vi "IT-M3900C List Output.vi"() -> ()   [LabVIEW 2015]
doc: "This example is used to edit the user - defined waveform function in source mode, call and implement the waveform output."
uses:
  <instrlib>/IT-M3900C/IT-M3900C.lvlib
panel:
  in  "Normal Voltage(V)":dbl min=0.0
  in  "Normal Current(A)":dbl
  in  "Serial Configuration":T1={"Baud Rate"=9600, "Parity"=0, "Data Bits"=8, "Stop Bits"=10, "Flow Control"=0} {"Flow Control" items=["None", "XON/XOFF", "RTS/CTS", "XON/XOFF & RTS/CTS", "DTR/DSR", "XON/XOFF & DTR/DSR"]; "Stop Bits" items=["1.0"=10, "1.5"=15, "2.0"=20]; "Data Bits" items=["7"=7, "8"=8]; "Parity" items=["None", "Odd", "Even", "Mark", "Space"]; "Baud Rate" items=["300"=300, "600"=600, "1200"=1200, "2400"=2400, "4800"=4800, "9600"=9600, "19200"=19200, "38400"=38400, "57600"=57600, "115200"=115200]}
  in  "Type":u16(ring) items=["Current", "Voltage"]
  in  "Save File(1-10)":i32=1 min=1 max=10
  in  "Terminate Type":u16(ring) items=["Normal", "Last", "Off"]
  in  "Repeat":i32 min=0
  in  "Slew":dbl[](array[numeric]) min=0.0
  in  "Dwell(S)":dbl[](array[numeric]) min=0.0
  in  "Level(V/A/W/ohm)":dbl[](array[numeric]) min=0.0
  in  "VISA resource name":refnum<visa-resource-name>
  # "List Function"
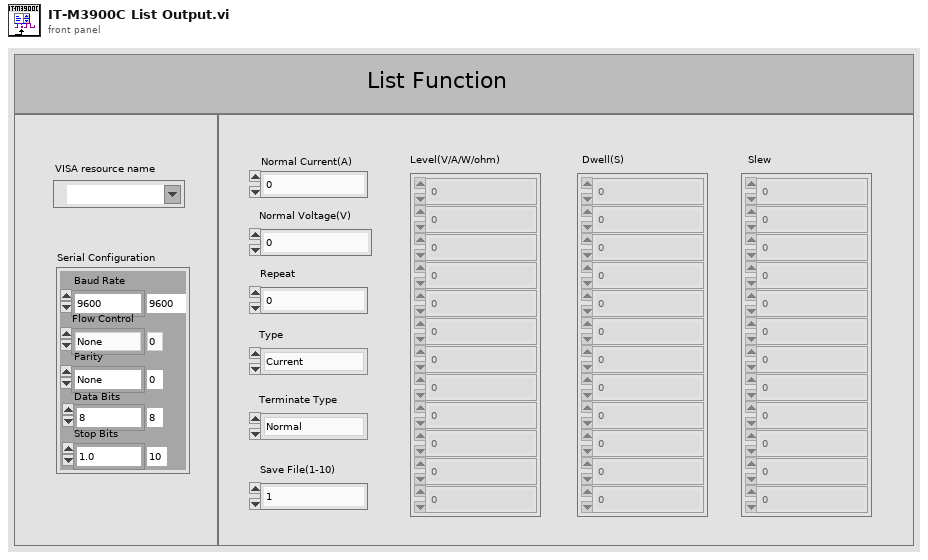
[diagram p1: front panel]
types:
  T1 = cluster{"Baud Rate":u32, "Parity":u16, "Data Bits":u16, "Stop Bits":u16, "Flow Control":u16}
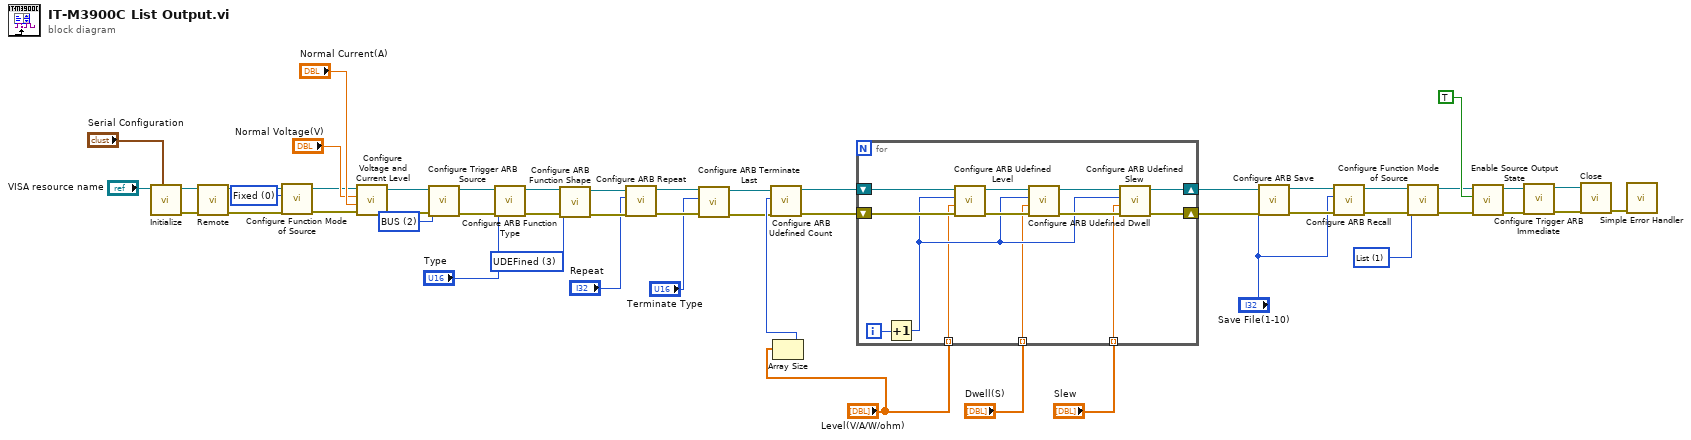
[diagram p0: block diagram]
diagram:
  w7 = u16 0 items=["Fixed", "List", "Battery", "Solar", "CarProfile", "Fuel", "Step"] ("Mode")
  w12 = u16 1 items=["Fixed", "List", "Battery", "Solar", "CarProfile", "Fuel", "Step"] ("Mode")
  w20 = u16 2 items=["IMMediate", "MANual", "BUS", "EXTernal"] ("Source")
  w38 = u16 3 items=["PULSe", "SINusiod", "SWEepsine", "UDEFined", "CDWell", "SEQuence"] ("Type")
  n1 = call <instrlib>:"Initialize.vi"("Serial Configuration"="Serial Configuration", "VISA resource name"="VISA resource name") -> ("error out"=w47:errorcluster, "VISA resource name out"=w48:refnum<visa-resource-name>)  [unwired: 8 in]
  n2 = call <instrlib>:"Remote.vi"("error in"=w47, "VISA resource name"=w48) -> ("error out"=w10:errorcluster, "VISA resource name out"=w11:refnum<visa-resource-name>)  [unwired: 8 in]
  n3 = call <instrlib>:"Configure Function Mode of Source.vi"("error in"=w10, "Mode"=w7, "VISA resource name"=w11) -> ("error out"=w9:errorcluster, "VISA resource name out"=w8:refnum<visa-resource-name>)  [unwired: 7 in]
  n4 = call <instrlib>:"Configure Voltage and Current Level.vi"("error in"=w9, "Current(A)"="Normal Current(A)", "Voltage(V)"="Normal Voltage(V)", "VISA resource name"=w8) -> ("error out"=w16:errorcluster, "VISA resource name out"=w15:refnum<visa-resource-name>)  [unwired: 6 in]
  n5 = call <instrlib>:"Configure Trigger ARB Source.vi"("error in"=w16, "Source"=w20, "VISA resource name"=w15) -> ("error out"=w22:errorcluster, "VISA resource name out"=w21:refnum<visa-resource-name>)  [unwired: 7 in]
  n6 = call <instrlib>:"Configure ARB Function Type.vi"("error in"=w22, "Type"="Type", "VISA resource name"=w21) -> ("error out"=w39:errorcluster, "VISA resource name out"=w40:refnum<visa-resource-name>)  [unwired: 7 in]
  n7 = call <instrlib>:"Configure ARB Function Shape.vi"("error in"=w39, "Type"=w38, "VISA resource name"=w40) -> ("error out"=w36:errorcluster, "VISA resource name out"=w37:refnum<visa-resource-name>)  [unwired: 7 in]
  n8 = call <instrlib>:"Configure ARB Repeat.vi"("error in"=w36, "Repeat"="Repeat", "VISA resource name"=w37) -> ("error out"=w33:errorcluster, "VISA resource name out"=w34:refnum<visa-resource-name>)  [unwired: 7 in]
  n9 = call <instrlib>:"Configure ARB Terminate Last.vi"("error in"=w33, "Type"="Terminate Type", "VISA resource name"=w34) -> ("error out"=w31:errorcluster, "VISA resource name out"=w32:refnum<visa-resource-name>)  [unwired: 7 in]
  n10 = Array Size(array="Level(V/A/W/ohm)") -> (size(s)=w43:i32)
  n11 = call <instrlib>:"Configure ARB Udefined Count.vi"("error in"=w31, "Count"=w43, "VISA resource name"=w32) -> ("error out"=w45:errorcluster, "VISA resource name out"=w46:refnum<visa-resource-name>)  [unwired: 7 in]
  n12 = for {
    shift-right: [w57] -> w29
    shift-left: w46 -> [w63]
    shift-right: [w56] -> w28
    shift-left: w45 -> [w62]
    tunnel: "Level(V/A/W/ohm)" -> [w53] mode=indexing
    tunnel: "Dwell(S)" -> [w52] mode=indexing
    tunnel: "Slew" -> [w51] mode=indexing
    i -> [w55]
    n13 = Increment(x=w55) -> (x+1=w54:i32)
    n14 = call <instrlib>:"Configure ARB Udefined Level.vi"("error in"=w62, "Level"=w53, "Step"=w54, "VISA resource name"=w63) -> ("error out"=w60:errorcluster, "VISA resource name out"=w61:refnum<visa-resource-name>)  [unwired: 6 in]
    n15 = call <instrlib>:"Configure ARB Udefined Dwell.vi"("error in"=w60, "DWELl"=w52, "Step"=w54, "VISA resource name"=w61) -> ("error out"=w58:errorcluster, "VISA resource name out"=w59:refnum<visa-resource-name>)  [unwired: 6 in]
    n16 = call <instrlib>:"Configure ARB Udefined Slew.vi"("error in"=w58, "Slew"=w51, "Step"=w54, "VISA resource name"=w59) -> ("error out"=w56:errorcluster, "VISA resource name out"=w57:refnum<visa-resource-name>)  [unwired: 6 in]
  }
  n17 = call <instrlib>:"Configure ARB Save.vi"("error in"=w28, "File"="Save File(1-10)", "VISA resource name"=w29) -> ("error out"=w27:errorcluster, "VISA resource name out"=w26:refnum<visa-resource-name>)  [unwired: 7 in]
  n18 = call <instrlib>:"Configure ARB Recall.vi"("error in"=w27, "File"="Save File(1-10)", "VISA resource name"=w26) -> ("error out"=w5:errorcluster, "VISA resource name out"=w6:refnum<visa-resource-name>)  [unwired: 7 in]
  n19 = call <instrlib>:"Configure Function Mode of Source.vi"("error in"=w5, "Mode"=w12, "VISA resource name"=w6) -> ("error out"=w3:errorcluster, "VISA resource name out"=w4:refnum<visa-resource-name>)  [unwired: 7 in]
  n20 = call <instrlib>:"Enable Source Output State.vi"("error in"=w3, "State"=TRUE, "VISA resource name"=w4) -> ("error out"=w2:errorcluster, "VISA resource name out"=w1:refnum<visa-resource-name>)  [unwired: 7 in]
  n21 = call <instrlib>:"Configure Trigger ARB Immediate.vi"("error in"=w2, "VISA resource name"=w1) -> ("error out"=w18:errorcluster, "VISA resource name out"=w19:refnum<visa-resource-name>)  [unwired: 8 in]
  n22 = call <instrlib>:"Close.vi"("error in"=w18, "VISA resource name"=w19) -> ("error out"=w49:errorcluster)  [unwired: 9 in]
  n23 = call <vilib>:"Simple Error Handler.vi"("error in (no error)"=w49) -> ()  [unwired: 4 in, 5 out]
